vi "Get Velocity Setpoint.vi"(8 "error in (no error)":errorcluster, 11 "simulated KUKA youBot wheel motor in":refnum<class "NI_Robotics_KUKA youBot Wheel Motor_Sim.lvclass">) -> (0 "error out":errorcluster, 2 "CCW velocity (rad/s)":dbl, 3 "simulated KUKA youBot wheel motor out":refnum<class "NI_Robotics_KUKA youBot Wheel Motor_Sim.lvclass">)   [LabVIEW 2017, in "NI_Robotics_KUKA youBot Host.lvlib" / "NI_Robotics_KUKA youBot Wheel Motor_Sim.lvclass"]
uses:
  <vilib>/robotics/KUKA youBot/Motor/Wheel Motor Sim/NI_Robotics_KUKA youBot Wheel Motor_Sim.lvclass
  <vilib>/robotics/KUKA youBot/Motor/Wheel Motor Sim/NI_Robotics_KUKA youBot Wheel Motor_Sim.lvclass/NI_Robotics_KUKA youBot Wheel Motor_Sim.ctl
  <vilib>/robotics/Simulator/Robot Factory/Motor/ODESimulator_Motor.lvclass
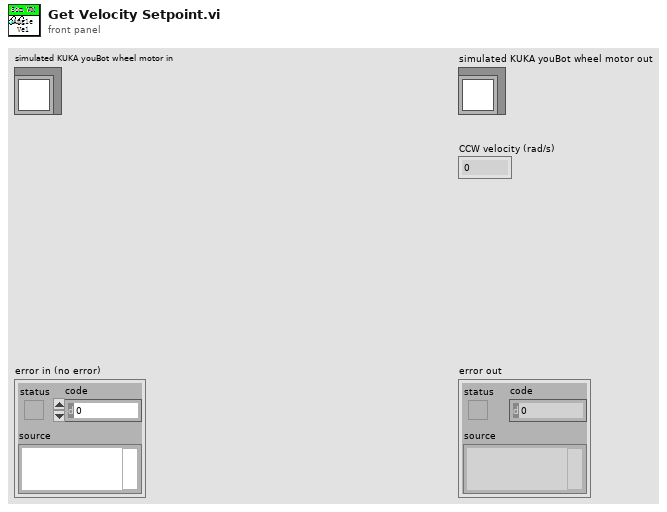
[diagram p1: front panel]
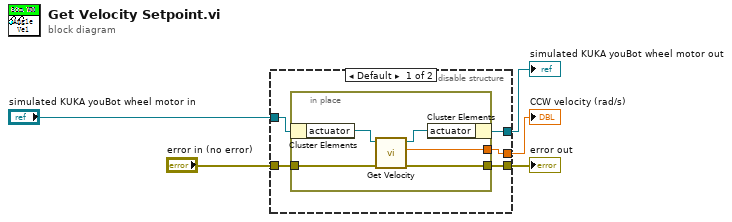
[diagram p0: block diagram]
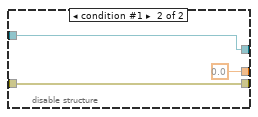
[diagram p2: hidden frame]
diagram:
  n1 = disable-structure shown="Default" {
    disable-tunnel: "simulated KUKA youBot wheel motor in" -> [w10 w18]
    disable-tunnel: [w9 w18] -> w3
    disable-tunnel: [w8 0.0 ("CCW Velocity (rad/s)")] -> w2
    disable-tunnel: "error in (no error)" -> [w7 w17]
    disable-tunnel: [w6 w17] -> w1
    frame condition #0 (active) {
      n2 = in-place {
        in-place-border: [w13] -> w8
        in-place-border: w7 -> [w12]
        in-place-border: [w11] -> w6
        n3 = in-place-cluster #1(w10) -> ("actuator"=w15:refnum<class "ODESimulator_Motor.lvclass">)
        n4 = call-dynamic "Get Velocity.vi"("error in (no error)"=w12, "Motor in"=w15) -> ("error out"=w11:errorcluster, "CCW Velocity (rad/s)"=w13:dbl, "Motor out"=w14:refnum<class "ODESimulator_Motor.lvclass">)  [unwired: 7 in]
        n5 = in-place-cluster #1("actuator"=w14) -> (w9:refnum<class "NI_Robotics_KUKA youBot Wheel Motor_Sim.lvclass">)
      }
    }
    frame condition #1 {
    }
  }
  "error out" <- w1
  "simulated KUKA youBot wheel motor out" <- w3
  "CCW velocity (rad/s)" <- w2
